vi "Typedef Default Value.vi"(7 "application reference (local)":refnum<vi>, 8 "error in (no error)":errorcluster, 11 "Name":string) -> (0 "error out":errorcluster, 3 "Value":variant)   [LabVIEW 2015, in "Scripting.lvlib"]
uses:
  Scripting.lvlib
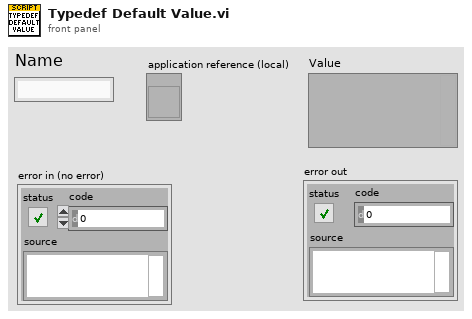
[diagram p1: front panel]
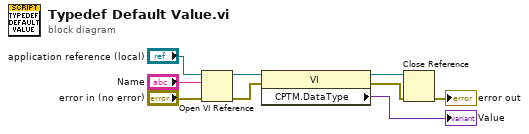
[diagram p0: block diagram]
diagram:
  n1 = Open VI Reference(application reference (local)="application reference (local)", vi path="Name", error in (no error)="error in (no error)") -> (vi reference=w8:refnum<vi>, error out=w6:errorcluster)  [unwired: 3 in]
  n2 = property class="VI"(reference=w8, error in=w6) -> (reference out=w7:refnum<vi>, error out=w5:errorcluster, "CPTM.DataType"=→"Value":variant)
  n3 = Close Reference(reference=w7, error in (no error)=w5) -> (error out=→"error out":errorcluster)
